vi "Add AIO Sections.vi"(8 "error in (no error)":errorcluster, 11 "Device Item Ref in":T1 format="%.0x") -> (0 "error out":errorcluster, 3 "Item Ref out":T1 format="%.0x")   [LabVIEW 2021, in "DAQ Analog InOut System Explorer.lvlib"]
uses:
  DAQ Analog InOut System Explorer.lvlib
  <vilib>/NI VeriStand/Custom Device API/Custom Device API.lvlib
  Shared/Constants.vi
  Shared/DAQ Analog InOut Shared.lvlib
  <vilib>/NI VeriStand/Custom Device API/Custom Device Item Ref.ctl
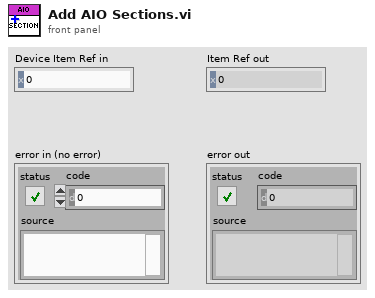
[diagram p1: front panel]
types:
  T1 = typedef "Custom Device API.lvlib/Custom Device Item Ref.ctl" = u64
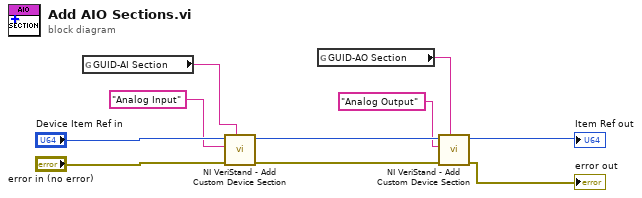
[diagram p0: block diagram]
diagram:
  n1 = global read "Constants.vi" "GUID-AI Section"() -> (w2:string)
  n2 = call <vilib>:"NI VeriStand - Add Custom Device Section.vi"("GUID (Default Section)"=w2, "error in (no error)"="error in (no error)", "Section Name"="Analog Input", "Parent Ref in"="Device Item Ref in") -> ("error out"=w6:errorcluster, "Parent Ref out"=w7:T1)  [unwired: 4 in, 2 out]
  n3 = global read "Constants.vi" "GUID-AO Section"() -> (w1:string)
  n4 = call <vilib>:"NI VeriStand - Add Custom Device Section.vi"("GUID (Default Section)"=w1, "error in (no error)"=w6, "Section Name"="Analog Output", "Parent Ref in"=w7) -> ("error out"=→"error out":errorcluster, "Parent Ref out"=→"Item Ref out":T1)  [unwired: 4 in, 2 out]
